vi "Logical Processors Used.vi"(4 "Set/Get (F)":bool, 5 "# Logical Processor Used":i32) -> (1 "# Logical Processor Used":i32)   [LabVIEW 2021, in "Utilities.lvlib"]
uses:
  Utilities.lvlib
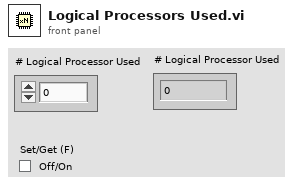
[diagram p1: front panel]
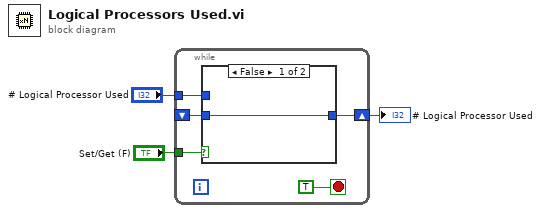
[diagram p0: block diagram]
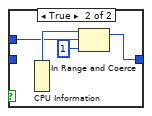
[diagram p2: hidden frame]
diagram:
  n1 = while {
    tunnel: "Set/Get (F)" -> [w7]
    shift-right: [w5] -> w1
    shift-left: _ -> [w4]
    tunnel: "# Logical Processor Used" -> [w6]
    stop <- TRUE stop-if-true
    n2 = case shown="False" w7 {
      tunnel: w6 -> [_ w12]
      tunnel: [w9 w10] -> w5
      tunnel: w4 -> [w9 _]
      frame False {
      }
      frame True {
        n3 = CPU Information() -> (4:w13:i32)  [unwired: 3 out]
        n4 = In Range and Coerce(upper limit=w13, x=w12, lower limit=1) -> (coerced(x)=w10:i32)  [unwired: 1 out]
      }
    }
  }
  "# Logical Processor Used" <- w1
